vi "OE_final_value.vi"(7 "time stamp":timestamp[](array[timestamp]), 11 "input cluster":T1={"connection reference"=refnum, "Net Avai time (Min)"=0, "pLAN dATE datA"=[], "Data by plan date, shift, product"=[], "BreakDownd Data"=[], "Raw rejection Data"=[], "mislanius times shift 1"={"Lunch Time From"=timestamp(3772857077 s since 1904-01-01), "Lunch Time To"=timestamp(3772857079 s since 1904-01-01), "Tea Time From"=timestamp(3772857095 s since 1904-01-01), "Tea Time To"=timestamp(3772857093 s since 1904-01-01), "Clean Time From"=timestamp(3772857086 s since 1904-01-01), "Clean Time To"=timestamp(3772857087 s since 1904-01-01), "Meeting Time From"=timestamp(3772857081 s since 1904-01-01), "Meeting Time To"=timestamp(3772857083 s since 1904-01-01), "Dev/Other Time From"=timestamp(3772857091 s since 1904-01-01), "Dev/Other Time To"=timestamp(3772857089 s since 1904-01-01), "Meeting"=TRUE, "Dev/Other"=TRUE}, "mislanius times shift 2"={"Lunch Time From"=timestamp(3772857057 s since 1904-01-01), "Lunch Time To"=timestamp(3772857059 s since 1904-01-01), "Tea Time From"=timestamp(3772857073 s since 1904-01-01), "Tea Time To"=timestamp(3772857072 s since 1904-01-01), "Clean Time From"=timestamp(3772857064 s since 1904-01-01), "Clean Time To"=timestamp(3772857066 s since 1904-01-01), "Meeting Time From"=timestamp(3772857061 s since 1904-01-01), "Meeting Time To"=timestamp(3772857063 s since 1904-01-01), "Dev/Other Time From"=timestamp(3772857070 s since 1904-01-01), "Dev/Other Time To"=timestamp(3772857068 s since 1904-01-01), "Meeting"=TRUE, "Dev/Other"=TRUE}} {"mislanius times shift 2"."Lunch Time From" format="%<%.X %x>T"; "mislanius times shift 2"."Lunch Time To" format="%<%.X %x>T"; "mislanius times shift 2"."Tea Time From" format="%<%.X %x>T"; "mislanius times shift 2"."Tea Time To" format="%<%.X %x>T"; "mislanius times shift 2"."Clean Time From" format="%<%.X %x>T"; "mislanius times shift 2"."Clean Time To" format="%<%.X %x>T"; "mislanius times shift 2"."Meeting Time From" format="%<%.X %x>T"; "mislanius times shift 2"."Meeting Time To" format="%<%.X %x>T"; "mislanius times shift 2"."Dev/Other Time From" format="%<%.X %x>T"; "mislanius times shift 2"."Dev/Other Time To" format="%<%.X %x>T"; "mislanius times shift 1"."Lunch Time From" format="%<%.X %x>T"; "mislanius times shift 1"."Lunch Time To" format="%<%.X %x>T"; "mislanius times shift 1"."Tea Time From" format="%<%.X %x>T"; "mislanius times shift 1"."Tea Time To" format="%<%.X %x>T"; "mislanius times shift 1"."Clean Time From" format="%<%.X %x>T"; "mislanius times shift 1"."Clean Time To" format="%<%.X %x>T"; "mislanius times shift 1"."Meeting Time From" format="%<%.X %x>T"; "mislanius times shift 1"."Meeting Time To" format="%<%.X %x>T"; "mislanius times shift 1"."Dev/Other Time From" format="%<%.X %x>T"; "mislanius times shift 1"."Dev/Other Time To" format="%<%.X %x>T"}) -> (1 "Breakdown time":u32, 2 "breakdown out time":string[](array[string]), 3 "breakdown in time":string[](array[string]))   [LabVIEW 2017]
uses:
  Controls/OE_screen_cluster.ctl
  <vilib>/addons/database/Connection.llb/Conn ObjectReference.ctl
  <vilib>/Utility/miscctls.llb/LVDateTimeRec.ctl
  <vilib>/addons/database/NI_Database_API.lvlib
panel:
  out "Breakdown Time":i32
  out "up time In Range?":bool
  out "down time In Range?":bool
  out "down time end":timestamp
  out "down time start":timestamp
  out "start time":timestamp
  out "end time":timestamp
  out "Start time":timestamp=timestamp(3772871939 s since 1904-01-01) format="%<%.X \n%x>T"
  out "End Time":timestamp=timestamp(3772871939 s since 1904-01-01) format="%<%.X \n%x>T"
  out "date time rec":T3
  in  "Cluster":T1={"connection reference"=refnum, "Net Avai time (Min)"=0, "pLAN dATE datA"=[], "Data by plan date, shift, product"=[], "BreakDownd Data"=[], "Raw rejection Data"=[], "mislanius times shift 1"={"Lunch Time From"=timestamp(0 s since 1904-01-01), "Lunch Time To"=timestamp(0 s since 1904-01-01), "Tea Time From"=timestamp(0 s since 1904-01-01), "Tea Time To"=timestamp(0 s since 1904-01-01), "Clean Time From"=timestamp(0 s since 1904-01-01), "Clean Time To"=timestamp(0 s since 1904-01-01), "Meeting Time From"=timestamp(0 s since 1904-01-01), "Meeting Time To"=timestamp(0 s since 1904-01-01), "Dev/Other Time From"=timestamp(0 s since 1904-01-01), "Dev/Other Time To"=timestamp(0 s since 1904-01-01), "Meeting"=FALSE, "Dev/Other"=TRUE}, "mislanius times shift 2"={"Lunch Time From"=timestamp(0 s since 1904-01-01), "Lunch Time To"=timestamp(0 s since 1904-01-01), "Tea Time From"=timestamp(0 s since 1904-01-01), "Tea Time To"=timestamp(0 s since 1904-01-01), "Clean Time From"=timestamp(0 s since 1904-01-01), "Clean Time To"=timestamp(0 s since 1904-01-01), "Meeting Time From"=timestamp(0 s since 1904-01-01), "Meeting Time To"=timestamp(0 s since 1904-01-01), "Dev/Other Time From"=timestamp(0 s since 1904-01-01), "Dev/Other Time To"=timestamp(0 s since 1904-01-01), "Meeting"=FALSE, "Dev/Other"=TRUE}} {"mislanius times shift 2"."Lunch Time From" format="%<%.X %x>T"; "mislanius times shift 2"."Lunch Time To" format="%<%.X %x>T"; "mislanius times shift 2"."Tea Time From" format="%<%.X %x>T"; "mislanius times shift 2"."Tea Time To" format="%<%.X %x>T"; "mislanius times shift 2"."Clean Time From" format="%<%.X %x>T"; "mislanius times shift 2"."Clean Time To" format="%<%.X %x>T"; "mislanius times shift 2"."Meeting Time From" format="%<%.X %x>T"; "mislanius times shift 2"."Meeting Time To" format="%<%.X %x>T"; "mislanius times shift 2"."Dev/Other Time From" format="%<%.X %x>T"; "mislanius times shift 2"."Dev/Other Time To" format="%<%.X %x>T"; "mislanius times shift 1"."Lunch Time From" format="%<%.X %x>T"; "mislanius times shift 1"."Lunch Time To" format="%<%.X %x>T"; "mislanius times shift 1"."Tea Time From" format="%<%.X %x>T"; "mislanius times shift 1"."Tea Time To" format="%<%.X %x>T"; "mislanius times shift 1"."Clean Time From" format="%<%.X %x>T"; "mislanius times shift 1"."Clean Time To" format="%<%.X %x>T"; "mislanius times shift 1"."Meeting Time From" format="%<%.X %x>T"; "mislanius times shift 1"."Meeting Time To" format="%<%.X %x>T"; "mislanius times shift 1"."Dev/Other Time From" format="%<%.X %x>T"; "mislanius times shift 1"."Dev/Other Time To" format="%<%.X %x>T"}
  in  "Select Product":string
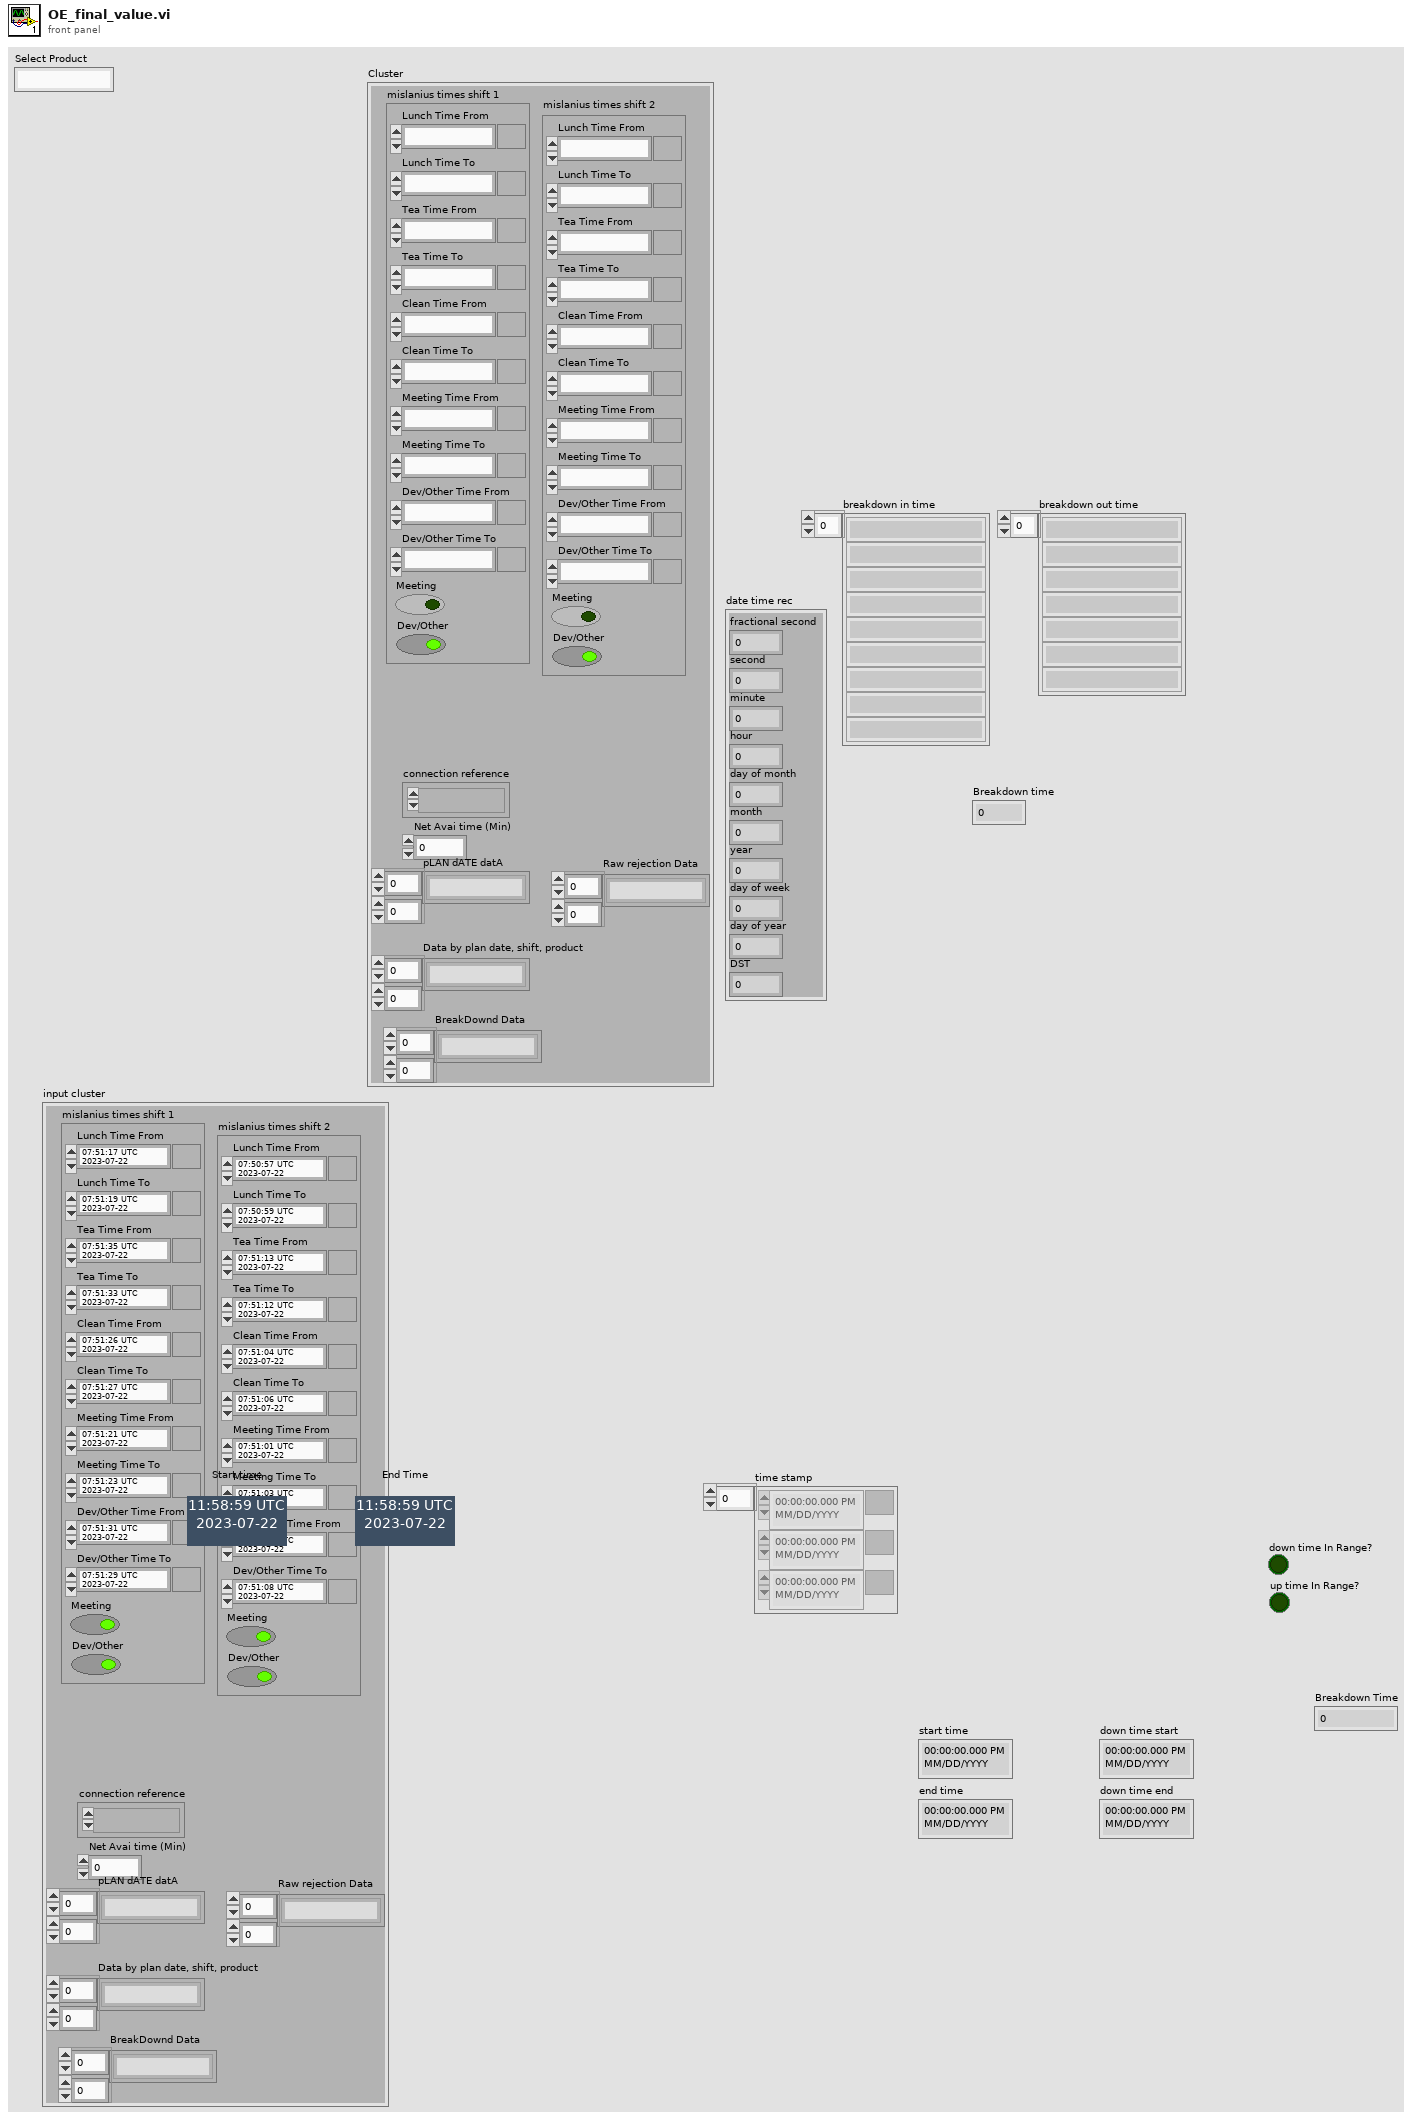
[diagram p1: front panel]
types:
  T1 = typedef "OE_screen_cluster.ctl" = cluster{"connection reference":T2, "Net Avai time (Min)":i32, "pLAN dATE datA":string[][], "Data by plan date, shift, product":string[][], "BreakDownd Data":string[][], "Raw rejection Data":string[][], "mislanius times shift 1":cluster{"Lunch Time From":timestamp, "Lunch Time To":timestamp, "Tea Time From":timestamp, "Tea Time To":timestamp, "Clean Time From":timestamp, "Clean Time To":timestamp, "Meeting Time From":timestamp, "Meeting Time To":timestamp, "Dev/Other Time From":timestamp, "Dev/Other Time To":timestamp, "Meeting":bool, "Dev/Other":bool}, "mislanius times shift 2":cluster{"Lunch Time From":timestamp, "Lunch Time To":timestamp, "Tea Time From":timestamp, "Tea Time To":timestamp, "Clean Time From":timestamp, "Clean Time To":timestamp, "Meeting Time From":timestamp, "Meeting Time To":timestamp, "Dev/Other Time From":timestamp, "Dev/Other Time To":timestamp, "Meeting":bool, "Dev/Other":bool}}
  T2 = typedef "NI_Database_API.lvlib/Conn ObjectReference.ctl" = refnum<k1>
  T3 = typedef "LVDateTimeRec.ctl" = cluster{"fractional second":dbl, "second":i32, "minute":i32, "hour":i32, "day of month":i32, "month":i32, "year":i32, "day of week":i32, "day of year":i32, "DST":i32}
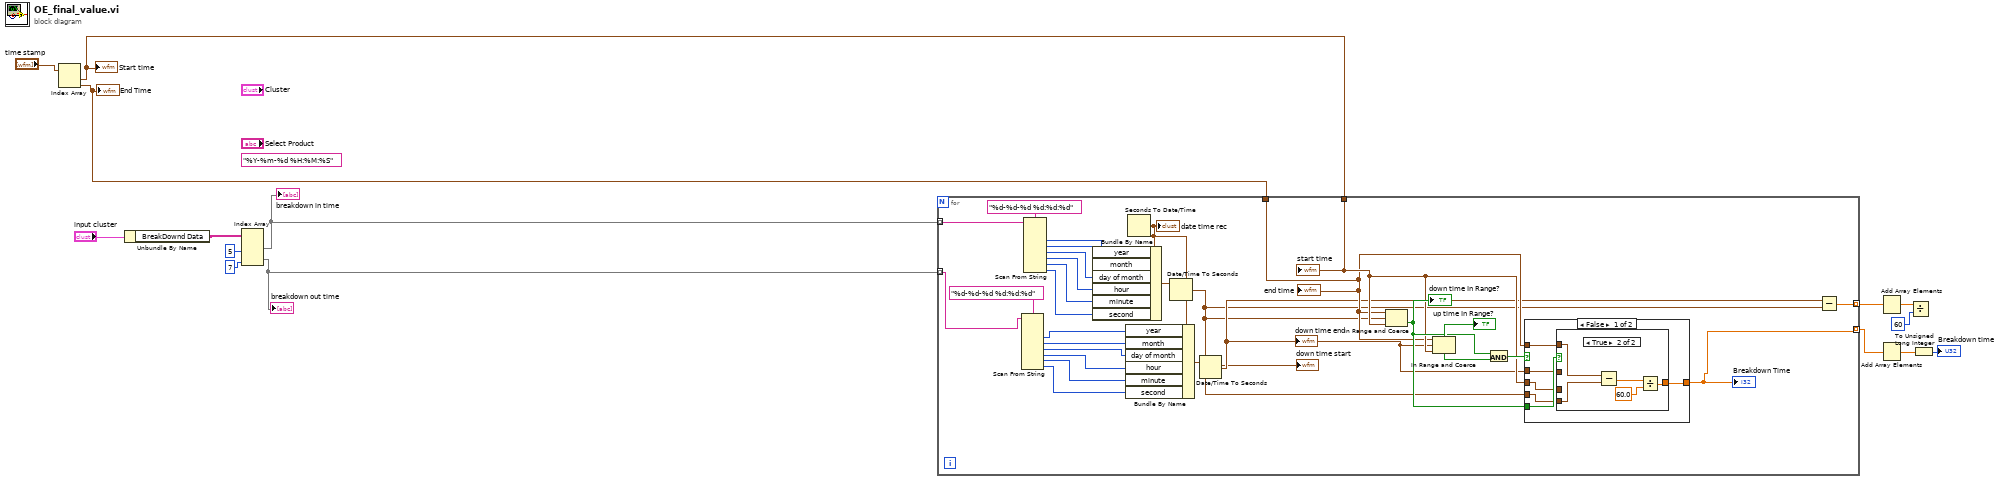
[diagram p0: block diagram]
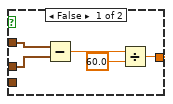
[diagram p2: hidden frame]
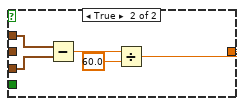
[diagram p3: hidden frame]
diagram:
  (unwired) "%Y-%m-%d %H:%M:%S" ("time format string (%c)")
  n1 = Index Array(array="time stamp") -> (element #1=w4:timestamp, element #2=w3:timestamp)  [unwired: 2 in]
  "End Time" <- w3
  "Start time" <- w4
  n2 = Unbundle By Name("input cluster") -> ("BreakDownd Data"=w7:string[][])
  n3 = Index Array(array=w7, index (col) #1=5 ("disabled index (col)"), index (col) #2=7 ("disabled index (col)")) -> (element #1=w13:string[], element #2=w12:string[])  [unwired: 2 in]
  "breakdown in time" <- w13
  "breakdown out time" <- w12
  n4 = for {
    tunnel: w13 -> [w42] mode=indexing
    tunnel: w12 -> [w28] mode=indexing
    tunnel: [w26] -> w11 mode=indexing
    tunnel: w4 -> [w20]
    tunnel: w3 -> [w19]
    tunnel: [w16] -> w2 mode=indexing
    n5 = Scan From String(format string="%d-%d-%d %d:%d:%d" ("time format string (%c)"), input string=w28) -> (output 1=w30:i32, output 2=w31:i32, output 3=w32:i32, output 4=w33:i32, output 5=w34:i32, output 6=w35:i32)  [unwired: 8 in, 3 out]
    n6 = Scan From String(format string="%d-%d-%d %d:%d:%d" ("time format string (%c)"), input string=w42) -> (output 1=w41:i32, output 2=w40:i32, output 3=w39:i32, output 4=w38:i32, output 5=w37:i32, output 6=w36:i32)  [unwired: 8 in, 3 out]
    n7 = Seconds To Date/Time() -> (date time rec=w27:T3)  [unwired: 2 in]
    "date time rec" <- w27
    n8 = Bundle By Name(cluster=w27, "year"=w41, "month"=w40, "day of month"=w39, "hour"=w38, "minute"=w37, "second"=w36) -> (w24:T3)
    n9 = Bundle By Name(cluster=w27, "year"=w30, "month"=w31, "day of month"=w32, "hour"=w33, "minute"=w34, "second"=w35) -> (w25:T3)
    n10 = Date/Time To Seconds(2:w24) -> (0:w17:timestamp)  [unwired: 1 in]
    "down time start" <- w17
    n11 = Date/Time To Seconds(2:w25) -> (0:w18:timestamp)  [unwired: 1 in]
    "down time end" <- w18
    n12 = In Range and Coerce(upper limit=w19, x=w17, lower limit=w20) -> (In Range?=w22:bool)  [unwired: 1 out]
    "down time In Range?" <- w22
    n13 = In Range and Coerce(upper limit=w19, x=w18, lower limit=w20) -> (In Range?=w23:bool)  [unwired: 1 out]
    "up time In Range?" <- w23
    n14 = And(x=w22, y=w23) -> (x .and. y?=w21:bool)
    n15 = case shown="False" w21 {
      tunnel: w22 -> [w49 _]
      tunnel: w20 -> [w48 _]
      tunnel: w18 -> [w47 w62]
      tunnel: [w46 w60] -> w16
      tunnel: w19 -> [w45 _]
      tunnel: w17 -> [w44 w61]
      frame False {
        n16 = case shown="True" w49 {
          tunnel: w48 -> [w54 _]
          tunnel: w47 -> [w53 _]
          tunnel: [w50 w55] -> w46
          tunnel: w45 -> [_ w57]
          tunnel: w44 -> [_ w56]
          frame False {
            n17 = Subtract(x=w53, y=w54) -> (x-y=w52:dbl)
            n18 = Divide(x=w52, y=60.0) -> (x/y=w50:dbl)
          }
          frame True {
            n19 = Subtract(x=w57, y=w56) -> (x-y=w59:dbl)
            n20 = Divide(x=w59, y=60.0) -> (x/y=w55:dbl)
          }
        }
      }
      frame True {
        n21 = Subtract(x=w62, y=w61) -> (x-y=w64:dbl)
        n22 = Divide(x=w64, y=60.0) -> (x/y=w60:dbl)
      }
    }
    "Breakdown Time" <- w16
    n23 = Subtract(x=w18, y=w17) -> (x-y=w26:dbl)
    "end time" <- w19
    "start time" <- w20
  }
  n24 = Add Array Elements(numeric array=w11) -> (sum=w8:dbl)
  n25 = Add Array Elements(numeric array=w2) -> (sum=w1:dbl)
  n26 = Divide(x=w8, y=60) -> ()  [unwired: 1 out]
  n27 = To Unsigned Long Integer(number=w1) -> (unsigned 32bit integer=→"Breakdown time":u32)
